vi "_Convert Model Name.vi"(2 "Model Name In":T1=enum."IONICS 3Q 210", 3 "Model":string) -> (0 "SingleSource":bool, 1 "Model Name":T1=enum."IONICS 3Q 210")   [LabVIEW 2015]
uses:
  Type/_Instrument Model.ctl
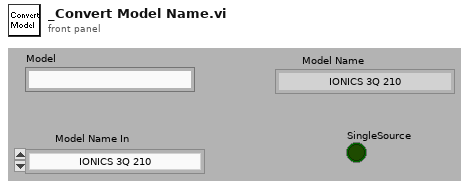
[diagram p1: front panel]
types:
  T1 = typedef "_Instrument Model.ctl" = enum16{"QSight 110", "QSight 120", "QSight 210", "QSight 220", "IONICS 3Q 110", "IONICS 3Q 120", "IONICS 3Q 210", "IONICS 3Q 220", "IONICS 3Q 310", "IONICS 3Q 320", "Simulation (Single Source)", "Simulation (Dual Source)"}
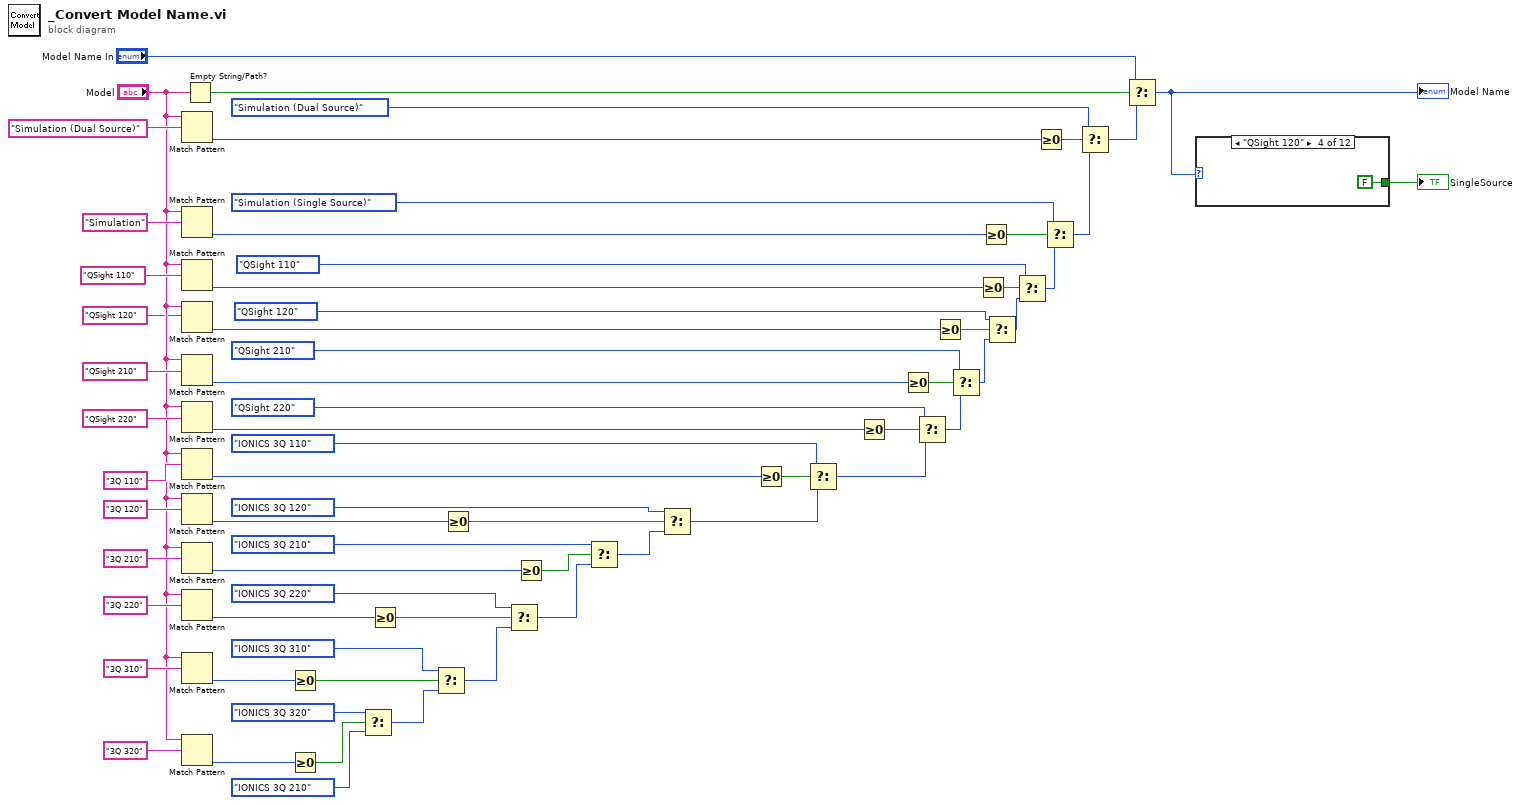
[diagram p0: block diagram]
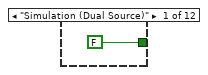
[diagram p2: hidden frame]
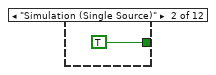
[diagram p3: hidden frame]
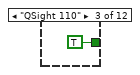
[diagram p4: hidden frame]
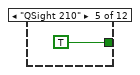
[diagram p5: hidden frame]
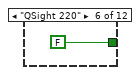
[diagram p6: hidden frame]
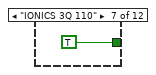
[diagram p7: hidden frame]
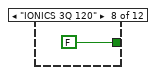
[diagram p8: hidden frame]
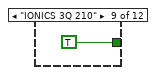
[diagram p9: hidden frame]
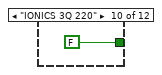
[diagram p10: hidden frame]
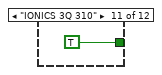
[diagram p11: hidden frame]
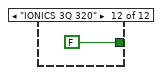
[diagram p12: hidden frame]
diagram:
  n1 = Match Pattern(string="Model", regular expression="Simulation (Dual Source)") -> (offset past match=w64:i32)  [unwired: 4 out]
  n2 = Match Pattern(string="Model", regular expression="Simulation") -> (offset past match=w49:i32)  [unwired: 4 out]
  n3 = Match Pattern(string="Model", regular expression="QSight 110") -> (offset past match=w8:i32)  [unwired: 4 out]
  n4 = Match Pattern(string="Model", regular expression="QSight 120") -> (offset past match=w9:i32)  [unwired: 4 out]
  n5 = Match Pattern(string="Model", regular expression="QSight 210") -> (offset past match=w54:i32)  [unwired: 4 out]
  n6 = Match Pattern(string="Model", regular expression="QSight 220") -> (offset past match=w55:i32)  [unwired: 4 out]
  n7 = Match Pattern(string="Model", regular expression="3Q 110") -> (offset past match=w47:i32)  [unwired: 4 out]
  n8 = Match Pattern(string="Model", regular expression="3Q 120") -> (offset past match=w48:i32)  [unwired: 4 out]
  n9 = Match Pattern(string="Model", regular expression="3Q 210") -> (offset past match=w39:i32)  [unwired: 4 out]
  n10 = Match Pattern(string="Model", regular expression="3Q 220") -> (offset past match=w17:i32)  [unwired: 4 out]
  n11 = Match Pattern(string="Model", regular expression="3Q 310") -> (offset past match=w20:i32)  [unwired: 4 out]
  n12 = Match Pattern(string="Model", regular expression="3Q 320") -> (offset past match=w21:i32)  [unwired: 4 out]
  n13 = Empty String/Path?(string/path="Model") -> (empty?=w29:bool)
  n14 = Greater Or Equal To 0?(x=w20) -> (x >= 0?=w19:bool)
  n15 = Greater Or Equal To 0?(x=w21) -> (x >= 0?=w22:bool)
  n16 = Select(t=_Instrument_Model."IONICS 3Q 320" ("Model Name"), s=w22, f=_Instrument_Model."IONICS 3Q 210" ("Model Name")) -> (s? t:f=w25:T1)
  n17 = Greater Or Equal To 0?(x=w17) -> (x >= 0?=w38:bool)
  n18 = Select(t=_Instrument_Model."IONICS 3Q 310" ("Model Name"), s=w19, f=w25) -> (s? t:f=w15:T1)
  n19 = Greater Or Equal To 0?(x=w48) -> (x >= 0?=w45:bool)
  n20 = Select(t=_Instrument_Model."IONICS 3Q 220" ("Model Name"), s=w38, f=w15) -> (s? t:f=w31:T1)
  n21 = Greater Or Equal To 0?(x=w39) -> (x >= 0?=w40:bool)
  n22 = Select(t=_Instrument_Model."IONICS 3Q 210" ("Model Name"), s=w40, f=w31) -> (s? t:f=w32:T1)
  n23 = Select(t=_Instrument_Model."IONICS 3Q 120" ("Model Name"), s=w45, f=w32) -> (s? t:f=w33:T1)
  n24 = Greater Or Equal To 0?(x=w47) -> (x >= 0?=w46:bool)
  n25 = Select(t=_Instrument_Model."IONICS 3Q 110" ("Model Name"), s=w46, f=w33) -> (s? t:f=w30:T1)
  n26 = Greater Or Equal To 0?(x=w55) -> (x >= 0?=w56:bool)
  n27 = Greater Or Equal To 0?(x=w54) -> (x >= 0?=w53:bool)
  n28 = Select(t=_Instrument_Model."QSight 220" ("Model Name"), s=w56, f=w30) -> (s? t:f=w62:T1)
  n29 = Greater Or Equal To 0?(x=w9) -> (x >= 0?=w6:bool)
  n30 = Select(t=_Instrument_Model."QSight 210" ("Model Name"), s=w53, f=w62) -> (s? t:f=w3:T1)
  n31 = Greater Or Equal To 0?(x=w8) -> (x >= 0?=w7:bool)
  n32 = Greater Or Equal To 0?(x=w49) -> (x >= 0?=w50:bool)
  n33 = Select(t=_Instrument_Model."QSight 120" ("Model Name"), s=w6, f=w3) -> (s? t:f=w2:T1)
  n34 = Select(t=_Instrument_Model."QSight 110" ("Model Name"), s=w7, f=w2) -> (s? t:f=w1:T1)
  n35 = Greater Or Equal To 0?(x=w64) -> (x >= 0?=w63:bool)
  n36 = Select(t=_Instrument_Model."Simulation (Single Source)" ("Model Name"), s=w50, f=w1) -> (s? t:f=w61:T1)
  n37 = Select(t=_Instrument_Model."Simulation (Dual Source)" ("Model Name"), s=w63, f=w61) -> (s? t:f=w27:T1)
  n38 = Select(t="Model Name In", s=w29, f=w27) -> (s? t:f=w14:T1)
  "Model Name" <- w14
  n39 = case shown="\"QSight 120\"" w14 {
    tunnel: [FALSE ("SingleSource") TRUE ("SingleSource") TRUE ("SingleSource") FALSE ("SingleSource") TRUE ("SingleSource") FALSE ("SingleSource") TRUE ("SingleSource") FALSE ("SingleSource") TRUE ("SingleSource") FALSE ("SingleSource") TRUE ("SingleSource") FALSE ("SingleSource")] -> w13
    frame "Simulation (Dual Source)" {
    }
    frame "Simulation (Single Source)" {
    }
    frame "QSight 110" {
    }
    frame "QSight 120" {
    }
    frame "QSight 210" {
    }
    frame "QSight 220" {
    }
    frame "IONICS 3Q 110" {
    }
    frame "IONICS 3Q 120" {
    }
    frame "IONICS 3Q 210" {
    }
    frame "IONICS 3Q 220" {
    }
    frame "IONICS 3Q 310" {
    }
    frame "IONICS 3Q 320" {
    }
  }
  "SingleSource" <- w13
